vi "Musictheory.vi"(2 "Numeric":dbl) -> (0 "Cluster":T1={"Keys"=["C", "C# / Db", "D", "D# / Eb", "E", "F", "F# / Gb", "G", "G# / Ab", "A", "A# / Bb", "B"], "Melodic Minor Scales"=["Melodic Minor", "Phrygian #6 (Dorian b2)", "Lydian Augmented", "Lydian Dominant (Mixolydian #4)", "Fifth Mode (Mixolydian b6, Hindu)", "Locrian #2 (Aeolian b5, Half Diminished)", "Altered (Diminished Whole Tone, Super Locrian)"], "Minor Tones"=[[TRUE, FALSE, TRUE, TRUE, FALSE, TRUE, FALSE, TRUE, FALSE, TRUE, FALSE, TRUE], [TRUE, TRUE, FALSE, TRUE, FALSE, TRUE, FALSE, TRUE, FALSE, TRUE, TRUE, FALSE], [TRUE, FALSE, TRUE, FALSE, TRUE, FALSE, TRUE, FALSE, TRUE, TRUE, FALSE, TRUE], [TRUE, FALSE, TRUE, FALSE, TRUE, FALSE, TRUE, TRUE, FALSE, TRUE, TRUE, FALSE], [TRUE, FALSE, TRUE, FALSE, TRUE, TRUE, FALSE, TRUE, TRUE, FALSE, TRUE, FALSE], [TRUE, FALSE, TRUE, TRUE, FALSE, TRUE, TRUE, FALSE, TRUE, FALSE, TRUE, FALSE], [TRUE, TRUE, FALSE, TRUE, TRUE, FALSE, TRUE, FALSE, TRUE, FALSE, TRUE, FALSE]], "Major Scales"=["Ionian (Major)", "Dorian", "Phrygian", "Lydian", "Mixolydian", "Aeolian (Natural/Pure Minor)", "Locrian"], "Major Tones"=[[TRUE, FALSE, TRUE, FALSE, TRUE, TRUE, FALSE, TRUE, FALSE, TRUE, FALSE, TRUE], [TRUE, FALSE, TRUE, TRUE, FALSE, TRUE, FALSE, TRUE, FALSE, TRUE, TRUE, FALSE], [TRUE, TRUE, FALSE, TRUE, FALSE, TRUE, FALSE, TRUE, TRUE, FALSE, TRUE, FALSE], [TRUE, FALSE, TRUE, FALSE, TRUE, FALSE, TRUE, TRUE, FALSE, TRUE, FALSE, TRUE], [TRUE, FALSE, TRUE, FALSE, TRUE, TRUE, FALSE, TRUE, FALSE, TRUE, TRUE, FALSE], [TRUE, FALSE, TRUE, TRUE, FALSE, TRUE, FALSE, TRUE, TRUE, FALSE, TRUE, FALSE], [TRUE, TRUE, FALSE, TRUE, FALSE, TRUE, TRUE, FALSE, TRUE, FALSE, TRUE, FALSE]], "Symmetric Scales"=["Whole Tone", "Diminished Whole Half (Whole Half)", "Diminished Half Whole (Half Whole)"], "Symmetric Tones"=[[TRUE, FALSE, TRUE, FALSE, TRUE, FALSE, TRUE, FALSE, TRUE, FALSE, TRUE, FALSE], [TRUE, FALSE, TRUE, TRUE, FALSE, TRUE, TRUE, FALSE, TRUE, TRUE, FALSE, TRUE], [TRUE, TRUE, FALSE, TRUE, TRUE, FALSE, TRUE, TRUE, FALSE, TRUE, TRUE, FALSE]], "Pentatonic Scales"=["Major Pentatonic", "Minor Pentatonic", "Suspended Pentatonic", "Dominant Pentatonic (Mixolydian Pentatonic)", "Traditional Japanese \"in sen\""], "Pentatonic Tones"=[[TRUE, FALSE, TRUE, FALSE, TRUE, FALSE, FALSE, TRUE, FALSE, TRUE, FALSE, FALSE], [TRUE, FALSE, FALSE, TRUE, FALSE, TRUE, FALSE, TRUE, FALSE, FALSE, TRUE, FALSE], [TRUE, FALSE, TRUE, FALSE, FALSE, TRUE, FALSE, TRUE, FALSE, FALSE, TRUE, FALSE], [TRUE, FALSE, TRUE, FALSE, TRUE, FALSE, FALSE, TRUE, FALSE, FALSE, TRUE, FALSE], [TRUE, TRUE, FALSE, FALSE, FALSE, TRUE, FALSE, TRUE, FALSE, FALSE, TRUE, FALSE]], "Blues Scale"=["Blues"], "Blues Tones"=[[TRUE, FALSE, FALSE, TRUE, FALSE, TRUE, TRUE, TRUE, FALSE, FALSE, TRUE, FALSE]], "Bebop Scale"=["Bebop Major", "Bebop Minor (Bebop Dorian)", "Bebop Dominant", "Bebop Melodic Minor"], "Bebop Tones"=[[TRUE, FALSE, TRUE, FALSE, TRUE, TRUE, FALSE, TRUE, TRUE, TRUE, FALSE, TRUE], [TRUE, FALSE, TRUE, TRUE, TRUE, TRUE, FALSE, TRUE, FALSE, TRUE, TRUE, FALSE], [TRUE, FALSE, TRUE, FALSE, TRUE, TRUE, FALSE, TRUE, FALSE, TRUE, TRUE, TRUE], [TRUE, FALSE, TRUE, TRUE, FALSE, TRUE, FALSE, TRUE, TRUE, TRUE, FALSE, TRUE]], "Harmonic Scales"=["Harmonic Major", "Harmonic Minor (Mohammedan)", "Double Harmonic Major (Arabic, Byzantine)"], "Harmonic Tones"=[[TRUE, FALSE, TRUE, FALSE, TRUE, TRUE, FALSE, TRUE, TRUE, FALSE, FALSE, TRUE], [TRUE, FALSE, TRUE, TRUE, FALSE, TRUE, FALSE, TRUE, TRUE, FALSE, FALSE, TRUE], [TRUE, TRUE, FALSE, FALSE, TRUE, TRUE, FALSE, TRUE, TRUE, FALSE, FALSE, TRUE]], "Exotic Scales"=["Hungarian Gypsy (Hungarian Minor)", "Hungarian Major", "Phrygian Dominant (Spanish, Spanish Phrygian, Spanish Gypsy, Jewish)", "Neapolitan Minor", "Neapolitan Major", "Enigmatic", "Eight-tone Spanish", "Balinese Pelog (Balinese, Pelog)", "Oriental", "Iwato", "Yo", "Promotheus", "Symmetrical", "Major Locrian (Arabian)"], "Exotic Tones"=[[TRUE, FALSE, TRUE, TRUE, FALSE, FALSE, TRUE, TRUE, TRUE, FALSE, FALSE, TRUE], [TRUE, FALSE, FALSE, TRUE, TRUE, FALSE, TRUE, TRUE, FALSE, TRUE, TRUE, FALSE], [TRUE, TRUE, FALSE, FALSE, TRUE, TRUE, FALSE, TRUE, TRUE, FALSE, TRUE, FALSE], [TRUE, TRUE, FALSE, TRUE, FALSE, TRUE, FALSE, TRUE, TRUE, FALSE, TRUE, TRUE], [TRUE, TRUE, FALSE, TRUE, FALSE, TRUE, FALSE, TRUE, FALSE, TRUE, FALSE, TRUE], [TRUE, TRUE, FALSE, FALSE, TRUE, FALSE, TRUE, FALSE, TRUE, FALSE, TRUE, TRUE], [TRUE, TRUE, FALSE, TRUE, TRUE, TRUE, TRUE, FALSE, TRUE, FALSE, TRUE, FALSE], [TRUE, TRUE, FALSE, TRUE, FALSE, FALSE, FALSE, TRUE, TRUE, FALSE, FALSE, FALSE], [TRUE, TRUE, FALSE, FALSE, TRUE, TRUE, TRUE, FALSE, FALSE, TRUE, TRUE, FALSE], [TRUE, TRUE, FALSE, FALSE, FALSE, TRUE, TRUE, FALSE, FALSE, FALSE, TRUE, FALSE], [TRUE, FALSE, TRUE, FALSE, FALSE, TRUE, FALSE, TRUE, FALSE, TRUE, FALSE, FALSE], [TRUE, FALSE, TRUE, FALSE, TRUE, FALSE, TRUE, FALSE, FALSE, TRUE, TRUE, FALSE], [TRUE, TRUE, FALSE, TRUE, FALSE, TRUE, FALSE, FALSE, TRUE, TRUE, TRUE, FALSE], [TRUE, FALSE, TRUE, FALSE, TRUE, TRUE, TRUE, FALSE, TRUE, FALSE, TRUE, FALSE]], "Miscellaneous Scales"=["Chromatic", "Augmented", "Lydian Minor"], "Miscellaneous Tones"=[[TRUE, TRUE, TRUE, TRUE, TRUE, TRUE, TRUE, TRUE, TRUE, TRUE, TRUE, TRUE], [TRUE, FALSE, FALSE, TRUE, TRUE, FALSE, FALSE, TRUE, TRUE, FALSE, FALSE, TRUE], [TRUE, FALSE, TRUE, FALSE, TRUE, FALSE, TRUE, TRUE, TRUE, FALSE, TRUE, FALSE]]})   [LabVIEW 2019]
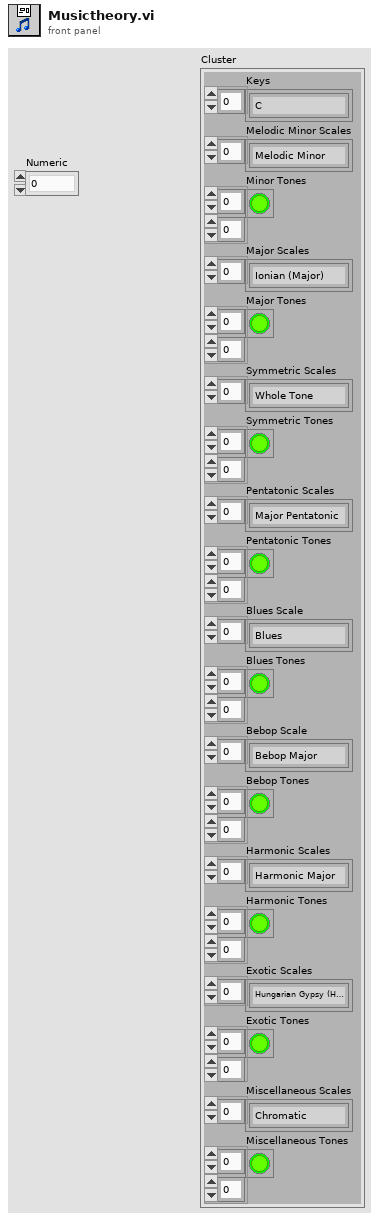
[diagram p1: front panel]
types:
  T1 = cluster{"Keys":string[], "Melodic Minor Scales":string[], "Minor Tones":bool[][], "Major Scales":string[], "Major Tones":bool[][], "Symmetric Scales":string[], "Symmetric Tones":bool[][], "Pentatonic Scales":string[], "Pentatonic Tones":bool[][], "Blues Scale":string[], "Blues Tones":bool[][], "Bebop Scale":string[], "Bebop Tones":bool[][], "Harmonic Scales":string[], "Harmonic Tones":bool[][], "Exotic Scales":string[], "Exotic Tones":bool[][], "Miscellaneous Scales":string[], "Miscellaneous Tones":bool[][]}
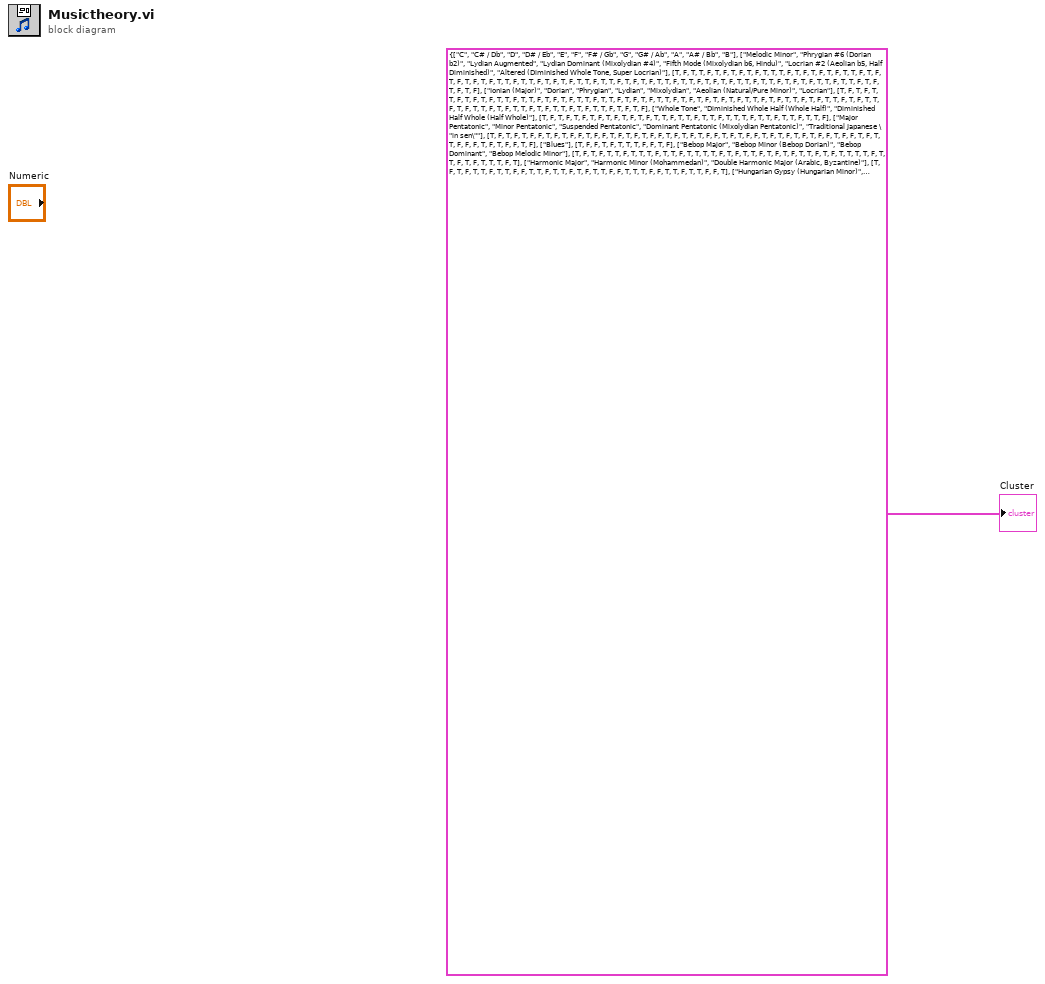
[diagram p0: block diagram]
diagram:
  "Cluster" <- T1 {"Keys"=["C", "C# / Db", "D", "D# / Eb", "E", "F", "F# / Gb", "G", "G# / Ab", "A", "A# / Bb", "B"], "Melodic Minor Scales"=["Melodic Minor", "Phrygian #6 (Dorian b2)", "Lydian Augmented", "Lydian Dominant (Mixolydian #4)", "Fifth Mode (Mixolydian b6, Hindu)", "Locrian #2 (Aeolian b5, Half Diminished)", "Altered (Diminished Whole Tone, Super Locrian)"], "Minor Tones"=[[TRUE, FALSE, TRUE, TRUE, FALSE, TRUE, FALSE, TRUE, FALSE, TRUE, FALSE, TRUE], [TRUE, TRUE, FALSE, TRUE, FALSE, TRUE, FALSE, TRUE, FALSE, TRUE, TRUE, FALSE], [TRUE, FALSE, TRUE, FALSE, TRUE, FALSE, TRUE, FALSE, TRUE, TRUE, FALSE, TRUE], [TRUE, FALSE, TRUE, FALSE, TRUE, FALSE, TRUE, TRUE, FALSE, TRUE, TRUE, FALSE], [TRUE, FALSE, TRUE, FALSE, TRUE, TRUE, FALSE, TRUE, TRUE, FALSE, TRUE, FALSE], [TRUE, FALSE, TRUE, TRUE, FALSE, TRUE, TRUE, FALSE, TRUE, FALSE, TRUE, FALSE], [TRUE, TRUE, FALSE, TRUE, TRUE, FALSE, TRUE, FALSE, TRUE, FALSE, TRUE, FALSE]], "Major Scales"=["Ionian (Major)", "Dorian", "Phrygian", "Lydian", "Mixolydian", "Aeolian (Natural/Pure Minor)", "Locrian"], "Major Tones"=[[TRUE, FALSE, TRUE, FALSE, TRUE, TRUE, FALSE, TRUE, FALSE, TRUE, FALSE, TRUE], [TRUE, FALSE, TRUE, TRUE, FALSE, TRUE, FALSE, TRUE, FALSE, TRUE, TRUE, FALSE], [TRUE, TRUE, FALSE, TRUE, FALSE, TRUE, FALSE, TRUE, TRUE, FALSE, TRUE, FALSE], [TRUE, FALSE, TRUE, FALSE, TRUE, FALSE, TRUE, TRUE, FALSE, TRUE, FALSE, TRUE], [TRUE, FALSE, TRUE, FALSE, TRUE, TRUE, FALSE, TRUE, FALSE, TRUE, TRUE, FALSE], [TRUE, FALSE, TRUE, TRUE, FALSE, TRUE, FALSE, TRUE, TRUE, FALSE, TRUE, FALSE], [TRUE, TRUE, FALSE, TRUE, FALSE, TRUE, TRUE, FALSE, TRUE, FALSE, TRUE, FALSE]], "Symmetric Scales"=["Whole Tone", "Diminished Whole Half (Whole Half)", "Diminished Half Whole (Half Whole)"], "Symmetric Tones"=[[TRUE, FALSE, TRUE, FALSE, TRUE, FALSE, TRUE, FALSE, TRUE, FALSE, TRUE, FALSE], [TRUE, FALSE, TRUE, TRUE, FALSE, TRUE, TRUE, FALSE, TRUE, TRUE, FALSE, TRUE], [TRUE, TRUE, FALSE, TRUE, TRUE, FALSE, TRUE, TRUE, FALSE, TRUE, TRUE, FALSE]], "Pentatonic Scales"=["Major Pentatonic", "Minor Pentatonic", "Suspended Pentatonic", "Dominant Pentatonic (Mixolydian Pentatonic)", "Traditional Japanese \"in sen\""], "Pentatonic Tones"=[[TRUE, FALSE, TRUE, FALSE, TRUE, FALSE, FALSE, TRUE, FALSE, TRUE, FALSE, FALSE], [TRUE, FALSE, FALSE, TRUE, FALSE, TRUE, FALSE, TRUE, FALSE, FALSE, TRUE, FALSE], [TRUE, FALSE, TRUE, FALSE, FALSE, TRUE, FALSE, TRUE, FALSE, FALSE, TRUE, FALSE], [TRUE, FALSE, TRUE, FALSE, TRUE, FALSE, FALSE, TRUE, FALSE, FALSE, TRUE, FALSE], [TRUE, TRUE, FALSE, FALSE, FALSE, TRUE, FALSE, TRUE, FALSE, FALSE, TRUE, FALSE]], "Blues Scale"=["Blues"], "Blues Tones"=[[TRUE, FALSE, FALSE, TRUE, FALSE, TRUE, TRUE, TRUE, FALSE, FALSE, TRUE, FALSE]], "Bebop Scale"=["Bebop Major", "Bebop Minor (Bebop Dorian)", "Bebop Dominant", "Bebop Melodic Minor"], "Bebop Tones"=[[TRUE, FALSE, TRUE, FALSE, TRUE, TRUE, FALSE, TRUE, TRUE, TRUE, FALSE, TRUE], [TRUE, FALSE, TRUE, TRUE, TRUE, TRUE, FALSE, TRUE, FALSE, TRUE, TRUE, FALSE], [TRUE, FALSE, TRUE, FALSE, TRUE, TRUE, FALSE, TRUE, FALSE, TRUE, TRUE, TRUE], [TRUE, FALSE, TRUE, TRUE, FALSE, TRUE, FALSE, TRUE, TRUE, TRUE, FALSE, TRUE]], "Harmonic Scales"=["Harmonic Major", "Harmonic Minor (Mohammedan)", "Double Harmonic Major (Arabic, Byzantine)"], "Harmonic Tones"=[[TRUE, FALSE, TRUE, FALSE, TRUE, TRUE, FALSE, TRUE, TRUE, FALSE, FALSE, TRUE], [TRUE, FALSE, TRUE, TRUE, FALSE, TRUE, FALSE, TRUE, TRUE, FALSE, FALSE, TRUE], [TRUE, TRUE, FALSE, FALSE, TRUE, TRUE, FALSE, TRUE, TRUE, FALSE, FALSE, TRUE]], "Exotic Scales"=["Hungarian Gypsy (Hungarian Minor)", "Hungarian Major", "Phrygian Dominant (Spanish, Spanish Phrygian, Spanish Gypsy, Jewish)", "Neapolitan Minor", "Neapolitan Major", "Enigmatic", "Eight-tone Spanish", "Balinese Pelog (Balinese, Pelog)", "Oriental", "Iwato", "Yo", "Promotheus", "Symmetrical", "Major Locrian (Arabian)"], "Exotic Tones"=[[TRUE, FALSE, TRUE, TRUE, FALSE, FALSE, TRUE, TRUE, TRUE, FALSE, FALSE, TRUE], [TRUE, FALSE, FALSE, TRUE, TRUE, FALSE, TRUE, TRUE, FALSE, TRUE, TRUE, FALSE], [TRUE, TRUE, FALSE, FALSE, TRUE, TRUE, FALSE, TRUE, TRUE, FALSE, TRUE, FALSE], [TRUE, TRUE, FALSE, TRUE, FALSE, TRUE, FALSE, TRUE, TRUE, FALSE, TRUE, TRUE], [TRUE, TRUE, FALSE, TRUE, FALSE, TRUE, FALSE, TRUE, FALSE, TRUE, FALSE, TRUE], [TRUE, TRUE, FALSE, FALSE, TRUE, FALSE, TRUE, FALSE, TRUE, FALSE, TRUE, TRUE], [TRUE, TRUE, FALSE, TRUE, TRUE, TRUE, TRUE, FALSE, TRUE, FALSE, TRUE, FALSE], [TRUE, TRUE, FALSE, TRUE, FALSE, FALSE, FALSE, TRUE, TRUE, FALSE, FALSE, FALSE], [TRUE, TRUE, FALSE, FALSE, TRUE, TRUE, TRUE, FALSE, FALSE, TRUE, TRUE, FALSE], [TRUE, TRUE, FALSE, FALSE, FALSE, TRUE, TRUE, FALSE, FALSE, FALSE, TRUE, FALSE], [TRUE, FALSE, TRUE, FALSE, FALSE, TRUE, FALSE, TRUE, FALSE, TRUE, FALSE, FALSE], [TRUE, FALSE, TRUE, FALSE, TRUE, FALSE, TRUE, FALSE, FALSE, TRUE, TRUE, FALSE], [TRUE, TRUE, FALSE, TRUE, FALSE, TRUE, FALSE, FALSE, TRUE, TRUE, TRUE, FALSE], [TRUE, FALSE, TRUE, FALSE, TRUE, TRUE, TRUE, FALSE, TRUE, FALSE, TRUE, FALSE]], "Miscellaneous Scales"=["Chromatic", "Augmented", "Lydian Minor"], "Miscellaneous Tones"=[[TRUE, TRUE, TRUE, TRUE, TRUE, TRUE, TRUE, TRUE, TRUE, TRUE, TRUE, TRUE], [TRUE, FALSE, FALSE, TRUE, TRUE, FALSE, FALSE, TRUE, TRUE, FALSE, FALSE, TRUE], [TRUE, FALSE, TRUE, FALSE, TRUE, FALSE, TRUE, TRUE, TRUE, FALSE, TRUE, FALSE]]}
